vi "SCMP - Run Cbk dispaly refesh.vi"(7 "mode":enum16{"Init", "Update", "Stop"}(ring)=enum."Update", 8 "error in (no error)":errorcluster, 9 "Cam idx":i32, 10 "Refresh Time {ms}":u32=1200) -> (0 "error out":errorcluster, 2 "Display Refresh":bool)   [LabVIEW 2014]
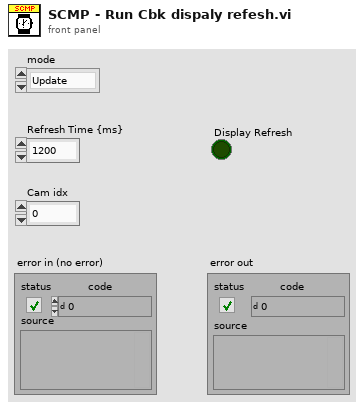
[diagram p1: front panel]
types:
  T1 = typedef "Semaphore RefNum" = refnum<k1>
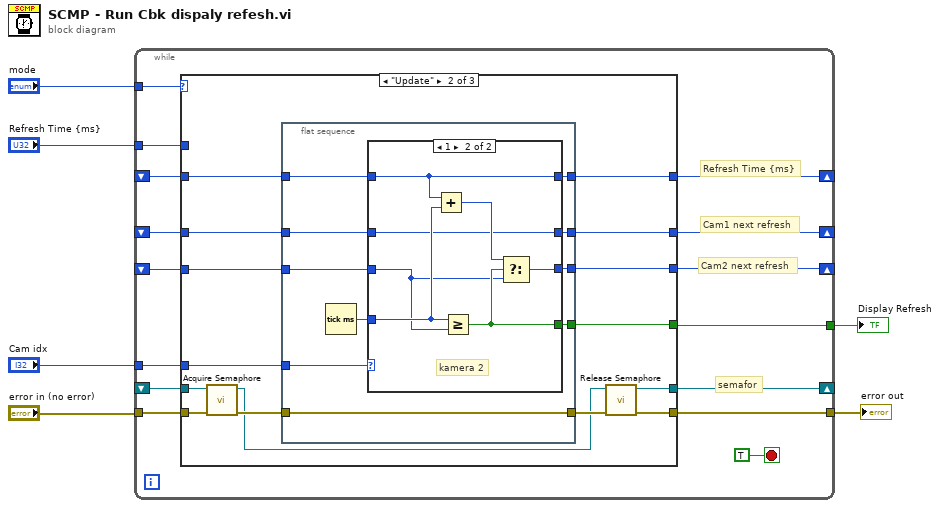
[diagram p0: block diagram]
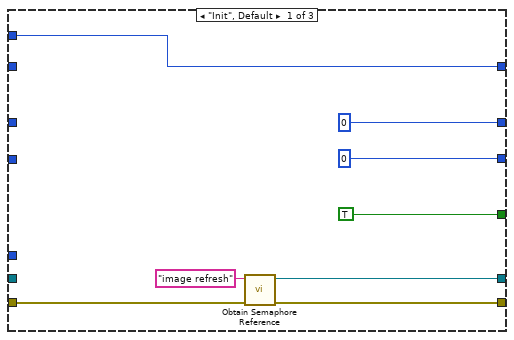
[diagram p2: hidden frame]
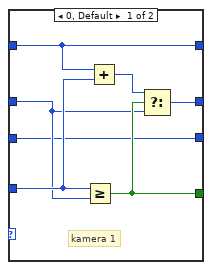
[diagram p3: hidden frame]
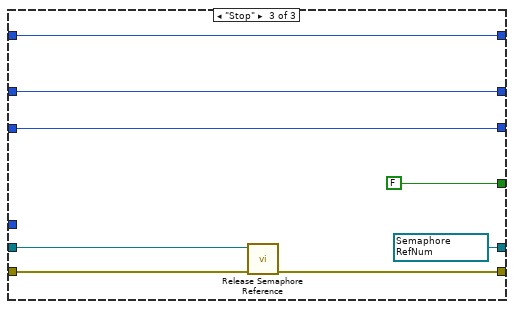
[diagram p4: hidden frame]
diagram:
  n1 = while {
    shift-right: [w21] -> _
    shift-left: _ -> [w14]
    tunnel: "Refresh Time {ms}" -> [w18]
    tunnel: "mode" -> [w19]
    shift-right: [w17] -> _
    shift-left: _ -> [w16]
    tunnel: [w15] -> w6
    tunnel: "Cam idx" -> [w13]
    shift-right: [w12] -> _
    shift-left: _ -> [w11]
    shift-right: [w7] -> _
    shift-left: _ -> [w10]
    tunnel: [w9] -> w1
    tunnel: "error in (no error)" -> [w8]
    stop <- TRUE stop-if-true
    # "semafor"
    # "Cam2 next refresh"
    # "Cam1 next refresh"
    # "Refresh Time {ms}"
    n2 = case shown="\"Update\"" w19 {
      tunnel: [TRUE w43 FALSE] -> w15
      tunnel: [u32 0 w41 w75] -> w21
      tunnel: w18 -> [w27 _ _]
      tunnel: [w27 w38 w74] -> w17
      tunnel: w16 -> [_ w44 w74]
      tunnel: w14 -> [_ w42 w75]
      tunnel: w13 -> [_ w40 _]
      tunnel: [u32 0 w37 w73] -> w12
      tunnel: w11 -> [_ w39 w73]
      tunnel: [w25 w31 w70] -> w7
      tunnel: w10 -> [_ w36 w69]
      tunnel: [w22 w32 w71] -> w9
      tunnel: w8 -> [w23 w34 w72]
      frame "Init", Default {
        n3 = call <vilib>:"Obtain Semaphore Reference.vi"("error in (no error)"=w23, "name (unnamed)"="image refresh") -> ("error out"=w22:errorcluster, "semaphore"=w25:T1)  [unwired: 3 in, 1 out]
      }
      frame "Update" {
        n4 = call <vilib>:"Acquire Semaphore.vi"("error in (no error)"=w34, "semaphore"=w36) -> ("error out"=w35:errorcluster, "semaphore out"=w30:T1)  [unwired: 3 in, 1 out]
        n5 = flat-sequence {
          tunnel: w44 -> [w54]
          tunnel: [w52] -> w43
          tunnel: w42 -> [w51]
          tunnel: [w50] -> w41
          tunnel: w40 -> [w49]
          tunnel: w39 -> [w48]
          tunnel: [w47] -> w38
          tunnel: [w46] -> w37
          tunnel: w35 -> [w45]
          tunnel: [w45] -> w33
          frame #0 {
            n6 = Tick Count (ms)() -> (millisecond timer value=w53:u32)
            n7 = case shown="1" w49 {
              tunnel: w54 -> [w56 w64]
              tunnel: w53 -> [w61 w68]
              tunnel: [w60 w67] -> w52
              tunnel: w51 -> [w59 w62]
              tunnel: [w57 w62] -> w50
              tunnel: w48 -> [w55 w65]
              tunnel: [w56 w64] -> w47
              tunnel: [w55 w63] -> w46
              frame 0, Default {
                # "kamera 1"
                n8 = Greater Or Equal?(x=w61, y=w59) -> (x >= y?=w60:bool)
                n9 = Add(x=w56, y=w61) -> (x+y=w58:u32)
                n10 = Select(t=w58, s=w60, f=w59) -> (s? t:f=w57:u32)
              }
              frame 1 {
                # "kamera 2"
                n11 = Add(x=w64, y=w68) -> (x+y=w66:u32)
                n12 = Greater Or Equal?(x=w68, y=w65) -> (x >= y?=w67:bool)
                n13 = Select(t=w66, s=w67, f=w65) -> (s? t:f=w63:u32)
              }
            }
          }
        }
        n14 = call <vilib>:"Release Semaphore.vi"("error in (no error)"=w33, "semaphore"=w30) -> ("error out"=w32:errorcluster, "semaphore out"=w31:T1)  [unwired: 4 in]
      }
      frame "Stop" {
        w70 = T1 refnum items=["semaphore"] ("semaphore out")
        n15 = call <vilib>:"Release Semaphore Reference.vi"("error in (no error)"=w72, "semaphore"=w69) -> ("error out"=w71:errorcluster)  [unwired: 8 in, 1 out]
      }
    }
  }
  "Display Refresh" <- w6
  "error out" <- w1
